vi "UDP 서버.vi"() -> ()   [LabVIEW 2018]
uses:
  <vilib>/Utility/tcp.llb/UDP Multicast Write-Only Open.vi
panel:
  out "날짜/시간 문자열":string
  in  "정지":bool
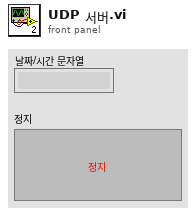
[diagram p1: front panel]
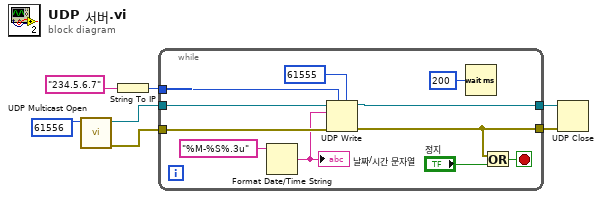
[diagram p0: block diagram]
diagram:
  n1 = call-poly <vilib>:"UDP Multicast Open.vi"("port"=u16 61556 ("포트")) -> ("error out"=w5:errorcluster, "connection ID"=w7:refnum<k16>)  [unwired: 9 in]
  n2 = String To IP(1:"234.5.6.7" ("이름")) -> (0:w2:u32)
  n3 = while {
    tunnel: w7 -> [w18]
    tunnel: [w17] -> w6
    tunnel: w5 -> [w16]
    tunnel: [w12] -> w4
    tunnel: w2 -> [w15]
    stop <- w11 stop-if-true
    n4 = Format Date/Time String(time format string (%c)="%M-%S%.3u" ("시간 포맷 문자열 (%c)")) -> (date/time string=w10:string)  [unwired: 2 in]
    "날짜/시간 문자열" <- w10
    n5 = UDP Write(address=w15, port or service name=u16 61555 ("포트 또는 서비스 이름"), connection ID=w18, data in=w10, 8:w16) -> (error out=w12:errorcluster, 3:w17:refnum<k16>)  [unwired: 1 in]
    n6 = Wait (ms)(milliseconds to wait=u32 200 ("대기 시간 (ms)")) -> ()  [unwired: 1 out]
    n7 = Or(x=w12, y="정지") -> (x .or. y?=w11:bool)
  }
  n8 = UDP Close(connection ID=w6, 8:w4) -> ()  [unwired: 2 out]
